vi "Flip (ARGB Both Axes).vi"(8 "error in (no error)":errorcluster, 10 "ARGB Destination Image":T1, 11 "ARGB Source Image":T1) -> (0 "error out":errorcluster, 3 "ARGB  Destination Image (duplicate)":T1)   [LabVIEW 2020, in "image.lvlib"]
uses:
  image.lvlib
  ARGB Image.ctl
  Flip Mode.ctl
  348de330-10c9-445f-8d54-7780e9118077.vi
  common/Module Path.vi
  <vilib>/Utility/error.llb/Error Cluster From Error Code.vi
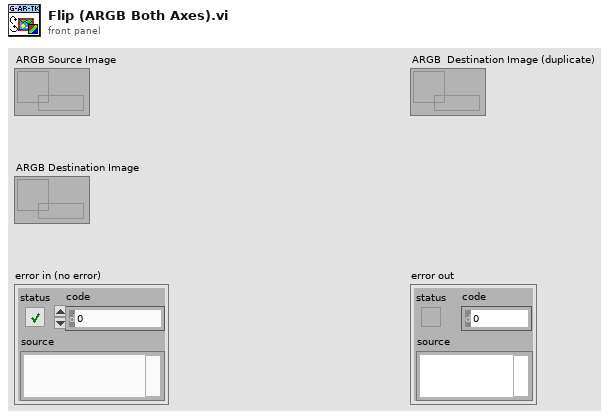
[diagram p1: front panel]
types:
  T1 = typedef "image.lvlib/ARGB Image.ctl" = refnum<data-value>
  T2 = typedef "image.lvlib/Flip Mode.ctl" = enum8{"X-Axis", "Y-Axis", "X and Y Axes"}
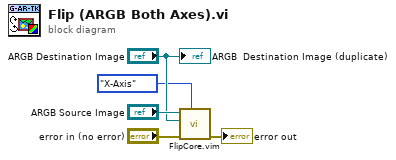
[diagram p0: block diagram]
diagram:
  n1 = call "FlipCore.vim"("Flip Mode"=Flip_Mode."X-Axis" ("Flip Mode (Default: Y-Axis)"), "error in (no error)"="error in (no error)", "Destination Image"="ARGB Destination Image", "Source Image"="ARGB Source Image") -> ("error out"=→"error out":errorcluster)  [unwired: 7 in]
  "ARGB  Destination Image (duplicate)" <- "ARGB Destination Image"
